vi "cv.to.local_team.vi"(8 "error in (no error)":errorcluster, 11 "cv team":T1) -> (0 "error out":errorcluster, 3 "local team":T5)   [LabVIEW 2024, in "CV_RESTful_Lib.lvlib"]
uses:
  CV_RESTful_Lib.lvlib
  <userlib>/_OpenG.lib/string/string.llb/openg_string.lvlib
  typedefs/local_team--cluster.ctl
  typedefs/cv_volume.publisher--cluster.ctl
  typedefs/cv_volume.issue--cluster.ctl
  typedefs/cv_team.results--cluster.ctl
  typedefs/cv_team--cluster.ctl
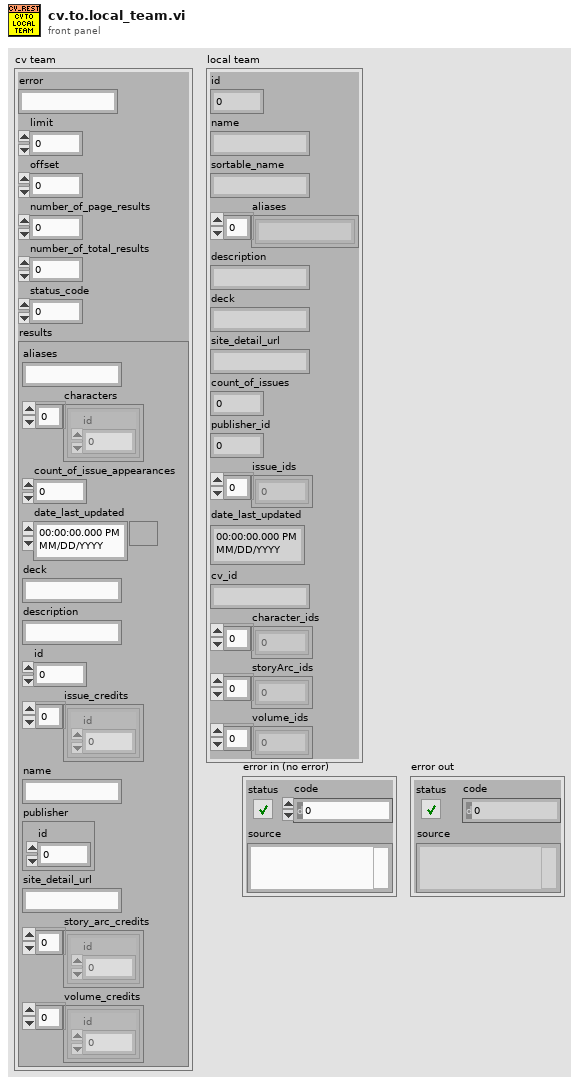
[diagram p1: front panel]
types:
  T1 = typedef "CV_RESTful_Lib.lvlib/cv_team--cluster.ctl" = cluster{"error":string, "limit":i32, "offset":i32, "number_of_page_results":i32, "number_of_total_results":i32, "status_code":i32, "results":T2}
  T2 = typedef "CV_RESTful_Lib.lvlib/cv_team.results--cluster.ctl" = cluster{"aliases":string, "characters":T3[], "count_of_issue_appearances":i32, "date_last_updated":timestamp, "deck":string, "description":string, "id":i32, "issue_credits":T3[], "name":string, "publisher":T4, "site_detail_url":string, "story_arc_credits":T3[], "volume_credits":T3[]}
  T3 = typedef "CV_RESTful_Lib.lvlib/cv_volume.issue--cluster.ctl" = cluster{"id":i32}
  T4 = typedef "CV_RESTful_Lib.lvlib/cv_volume.publisher--cluster.ctl" = cluster{"id":i32}
  T5 = typedef "CV_RESTful_Lib.lvlib/local_team--cluster.ctl" = cluster{"id":i32, "name":string, "sortable_name":string, "aliases":string[], "description":string, "deck":string, "site_detail_url":string, "count_of_issues":i32, "publisher_id":i32, "issue_ids":i32[], "date_last_updated":timestamp, "cv_id":string, "character_ids":i32[], "storyArc_ids":i32[], "volume_ids":i32[]}
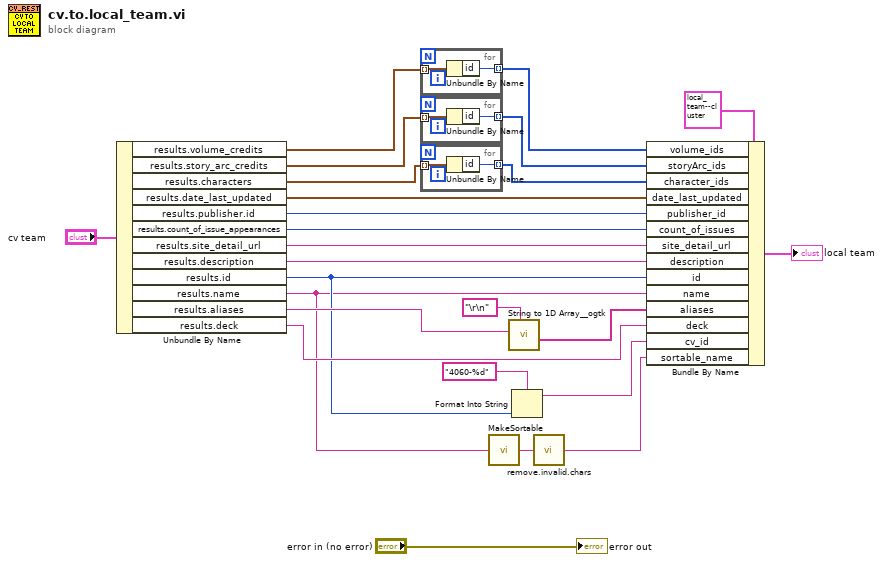
[diagram p0: block diagram]
diagram:
  n1 = Unbundle By Name("cv team") -> ("results.volume_credits"=w4:T3[], "results.story_arc_credits"=w5:T3[], "results.characters"=w6:T3[], "results.date_last_updated"=w7:timestamp, "results.publisher.id"=w15:i32, "results.count_of_issue_appearances"=w16:i32, "results.site_detail_url"=w17:string, "results.description"=w18:string, "results.id"=w12:i32, "results.name"=w9:string, "results.aliases"=w21:string, "results.deck"=w14:string)
  n2 = for {
    tunnel: w4 -> [w27] mode=indexing
    tunnel: [w26] -> w1 mode=indexing
    n3 = Unbundle By Name(w27) -> ("id"=w26:i32)
  }
  n4 = for {
    tunnel: w5 -> [w29] mode=indexing
    tunnel: [w28] -> w2 mode=indexing
    n5 = Unbundle By Name(w29) -> ("id"=w28:i32)
  }
  n6 = for {
    tunnel: w6 -> [w31] mode=indexing
    tunnel: [w30] -> w3 mode=indexing
    n7 = Unbundle By Name(w31) -> ("id"=w30:i32)
  }
  n8 = call "MakeSortable.vi"("string in"=w9) -> ("string out"=w22:string)
  n9 = call <userlib>:"String to 1D Array__ogtk.vi"("delimiter (Tab)"="\r\n", "string"=w21) -> ("Array of Strings"=w19:string[])  [unwired: 9 in]
  n10 = Format Into String(format string="4060-%d", w12) -> (resulting string=w11:string)  [unwired: 2 in, 1 out]
  n11 = call "remove.invalid.chars.vi"("string in"=w22) -> ("string out"=w8:string)
  n12 = Bundle By Name(cluster=T5 {"id"=0, "name"="", "sortable_name"="", "aliases"=[], "description"="", "deck"="", "site_detail_url"="", "count_of_issues"=0, "publisher_id"=0, "issue_ids"=[], "date_last_updated"=timestamp(0 s since 1904-01-01), "cv_id"="", "character_ids"=[], "storyArc_ids"=[], "volume_ids"=[]} ("local team"), "volume_ids"=w1, "storyArc_ids"=w2, "character_ids"=w3, "date_last_updated"=w7, "publisher_id"=w15, "count_of_issues"=w16, "site_detail_url"=w17, "description"=w18, "id"=w12, "name"=w9, "aliases"=w19, "deck"=w14, "cv_id"=w11, "sortable_name"=w8) -> (→"local team":T5)
  "error out" <- "error in (no error)"
